vi "Delete Temp File.vi"(8 "error in":errorcluster, 11 "file path in":path) -> (0 "error out":errorcluster)   [LabVIEW 2019]
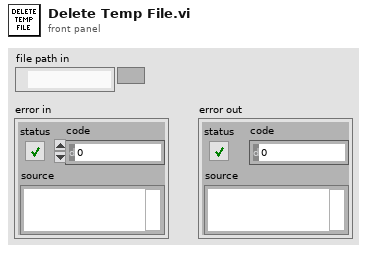
[diagram p1: front panel]
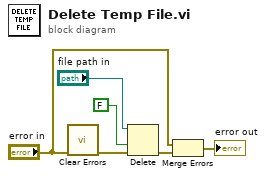
[diagram p0: block diagram]
diagram:
  n1 = call <vilib>:"Clear Errors.vi"("error in (no error)"="error in") -> ("error out"=w4:errorcluster)  [unwired: 5 in, 1 out]
  n2 = Delete(path (use dialog)="file path in", confirm (F)=FALSE, error in=w4) -> (error out=w2:errorcluster)  [unwired: 2 in, 2 out]
  n3 = Merge Errors("error in", w2) -> (→"error out":errorcluster)
